vi "GetAcquisitionTimingsSD.vi"(0 "exposure input":sgl format="%.2f", 5 "accumulate input":sgl format="%.2f", 7 "kinetic input":sgl format="%.2f", 11 "error in (no error)":errorcluster) -> (4 "exposure":sgl format="%.2f", 6 "accumulate":sgl format="%.2f", 8 "kinetic":sgl format="%.2f", 10 "DLL error code":u32, 15 "error out":errorcluster)   [LabVIEW 2015]
doc: "This function will return the current \"valid\" acquisition timing information. This function should be used after all the acquisitions settings have been set, e.g. <B>SetExposureTime</B>, <B>SetKineticCycleTime</B> and <B>SetReadMode</B> etc. The values returned are the actual times used in subsequent acquisitions.\n\nThis function is required as it is possible to set the exposure time to 20ms, accumulate cycle time to 30ms and then set the read out mode to full image. As it can take 250ms to read out an image it is not possible to have a cycle time of 30ms.\n\n<B>Parameters:</B>\nexposure - valid exposure time in seconds\naccumulate - valid accumulate cycle time in seconds\nkinetic - valid kinetic cycle time in seconds\n\n<B>Error codes:</B>\nDRV_SUCCESS - Timing information returned.\nDRV_NOT_INITIALIZED - System not initialized.\nDRV_ACQUIRING - Acquisition in progress.\nDRV_INVALID_MODE - Acquisition or readout mode is not available."
uses:
  DLL/atmcd32d.dll
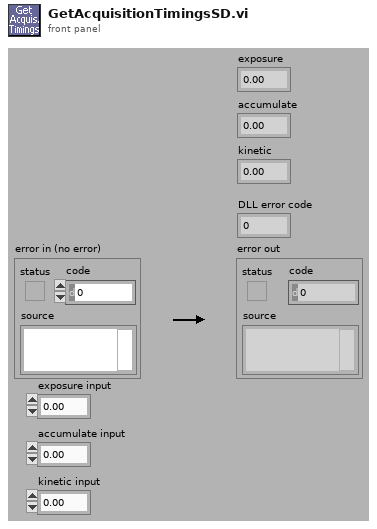
[diagram p1: front panel]
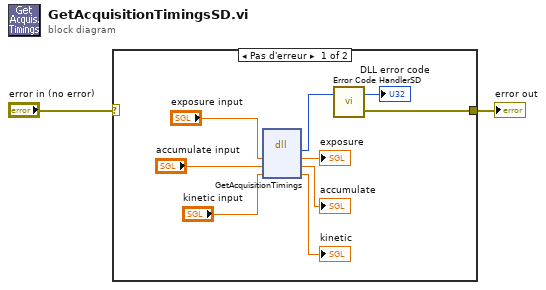
[diagram p0: block diagram]
diagram:
  n1 = case shown="Pas d'erreur" "error in (no error)" {
    selector: "error in (no error)" -> [_ w12]
    tunnel: [w10 w12] -> w1
    frame No Error {
      n2 = dll-call lib="G:/SD/TRANCON-2015/DLL/Atmcd32d.dll" fn="GetAcquisitionTimings"("exposure"="exposure input", "accumulate"="accumulate input", "kinetic"="kinetic input") -> (w11:u32, "exposure"=→"exposure":sgl, "accumulate"=→"accumulate":sgl, "kinetic"=→"kinetic":sgl)  [unwired: 3 in, 2 out]
      n3 = call "Error Code HandlerSD.vi"("DLL error code"=w11) -> ("error out"=w10:errorcluster, "dup DLL error code"=→"DLL error code":u32)  [unwired: 1 in]
    }
    frame Error {
    }
  }
  "error out" <- w1
